vi "Configure Number of Points.vi"(8 "error in (no error)":errorcluster, 10 "Number of Point":i32, 11 "VNA-FieldFox in":refnum<class "VNA-FieldFox.lvclass">) -> (0 "error out":errorcluster, 3 "VNA-FieldFox out":refnum<class "VNA-FieldFox.lvclass">)   [LabVIEW 2020, in "VNA-FieldFox.lvclass"]
doc: "Configures the number of points in the sweep.\nThe number of points will be choosen to the nearest supported."
uses:
  VNA-FieldFox.lvclass
  C:/Sandbox/RF Bench/Source Code/WiSpry Test Framework/Instruments/Instrument.lvclass
  C:/Sandbox/RF Bench/Source Code/WiSpry Test Framework/Instruments/Vector Network Analyzer/Vector Network Analyzer.lvclass
  Instrument.lvclass/Instrument.ctl
  Vector Network Analyzer.lvclass/Vector Network Analyzer.ctl
  <instrlib>/Agilent N99XX Series/Agilent N99XX Series.lvlib
  Instrument.lvclass
  Vector Network Analyzer.lvclass
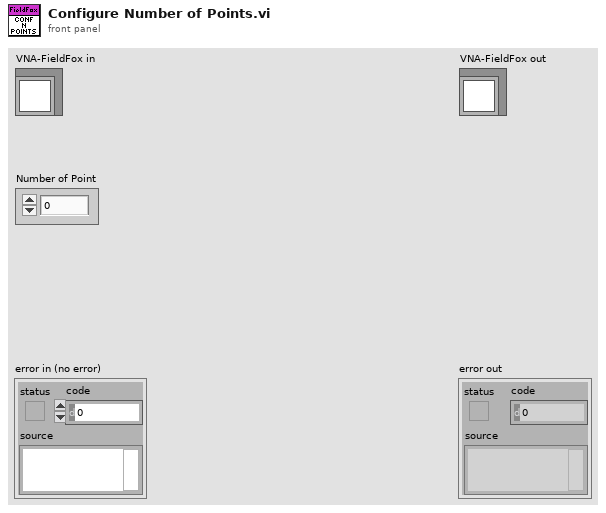
[diagram p1: front panel]
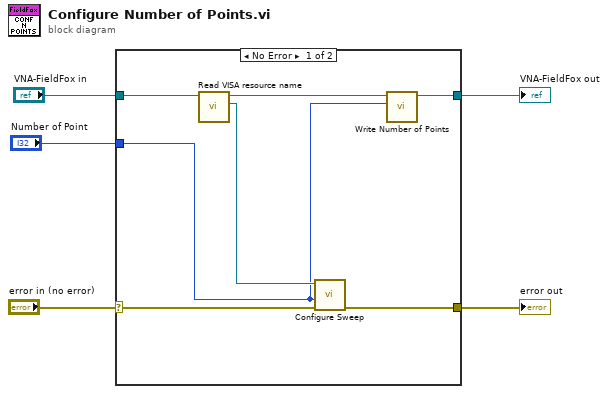
[diagram p0: block diagram]
diagram:
  n1 = case shown="No Error" "error in (no error)" {
    selector: "error in (no error)" -> [w10 w14]
    tunnel: "VNA-FieldFox in" -> [w12 w13]
    tunnel: "Number of Point" -> [w8 _]
    tunnel: [w9 w14] -> w2
    tunnel: [w6 w13] -> w1
    frame No Error {
      n2 = call "Read VISA resource name.vi"("Instrument in"=w12) -> ("VISA resource name"=w11:refnum<visa-resource-name>, "Instrument out"=w7:refnum<class "VNA-FieldFox.lvclass">)  [unwired: 9 in]
      n3 = call <instrlib>:"Configure Sweep.vi"("error in (no error)"=w10, "Data Point (401)"=w8, "VISA resource name"=w11) -> ("error out"=w9:errorcluster)  [unwired: 7 in, 1 out]
      n4 = call "Write Number of Points.vi"("Number of Points"=w8, "Vector Network Analyzer in"=w7) -> ("Vector Network Analyzer out"=w6:refnum<class "VNA-FieldFox.lvclass">)  [unwired: 9 in]
    }
    frame Error {
    }
  }
  "error out" <- w2
  "VNA-FieldFox out" <- w1
